vi "Time Target Completed.vi"(10 "Step Status":string, 11 "Time Completed?":bool) -> (3 "Machine State":T1(ring))   [LabVIEW 2020]
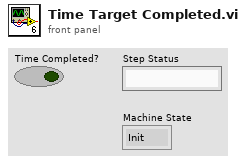
[diagram p1: front panel]
types:
  T1 = enum16{"Init", "Wait to Start", "Step In Progress", "Next Step", "Wait Fix Position"}
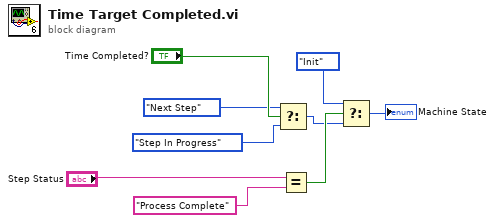
[diagram p0: block diagram]
diagram:
  n1 = Select(t=T1."Next Step" ("Machine States"), s="Time Completed?", f=T1."Step In Progress" ("Machine States")) -> (s? t:f=w2:T1)
  n2 = Equal?(x="Step Status", y="Process Complete") -> (x = y?=w3:bool)
  n3 = Select(t=T1."Init", s=w3, f=w2) -> (s? t:f=→"Machine State":T1)
